vi "xijk_error clean up.vi"(8 "error in":errorcluster, 11 "code in":i32) -> (0 "error out":errorcluster)   [LabVIEW 2009]
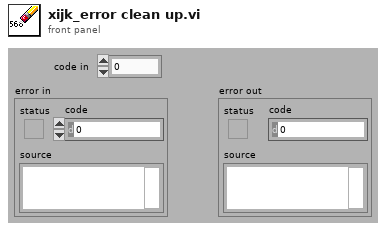
[diagram p1: front panel]
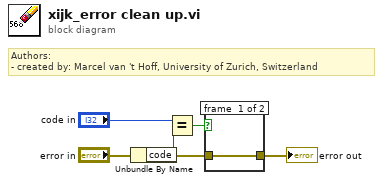
[diagram p0: block diagram]
diagram:
  # "Authors: \n- created by: Marcel van 't Hoff, University of Zurich, Switzerland"
  n1 = Unbundle By Name("error in") -> ("code"=w5:i32)
  n2 = Equal?(x="code in", y=w5) -> (x = y?=w1:bool)
  n3 = case shown="False" w1 {
    tunnel: [w6 _] -> w3
    tunnel: "error in" -> [w6 _]
    frame #0 {
    }
    frame #1 {
    }
  }
  "error out" <- w3
